vi "XYStage.KIM101.Create Device.vi"(8 "error in (no error)":errorcluster, 11 "SerialNumber":string="97000001") -> (0 "error out":errorcluster, 2 "Device":refnum<k24>, 3 "KCubeInertialMotorControl":refnum<k24>, 5 "CreateDevice Result":bool)   [LabVIEW 2017, in "XYStage.KIM101.lvclass"]
uses:
  XYStage.KIM101.lvclass
  D:/upwork/Laser Measurement Tool/Laser/project/data/Thorlabs.MotionControl.Controls.dll
  data/Thorlabs.MotionControl.Controls.dll
  D:/upwork/Laser Measurement Tool/Laser/project/data/Thorlabs.MotionControl.KCube.InertialMotorCLI.dll
  data/Thorlabs.MotionControl.KCube.InertialMotorCLI.dll
panel:
  in  "KCubeInertialMotorControl":refnum<k24>(container)
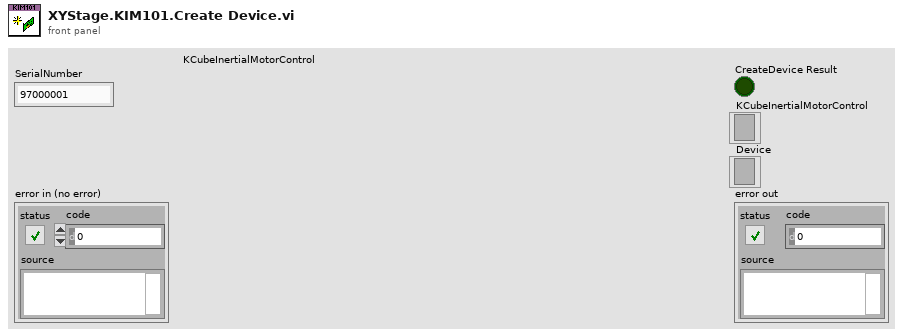
[diagram p1: front panel]
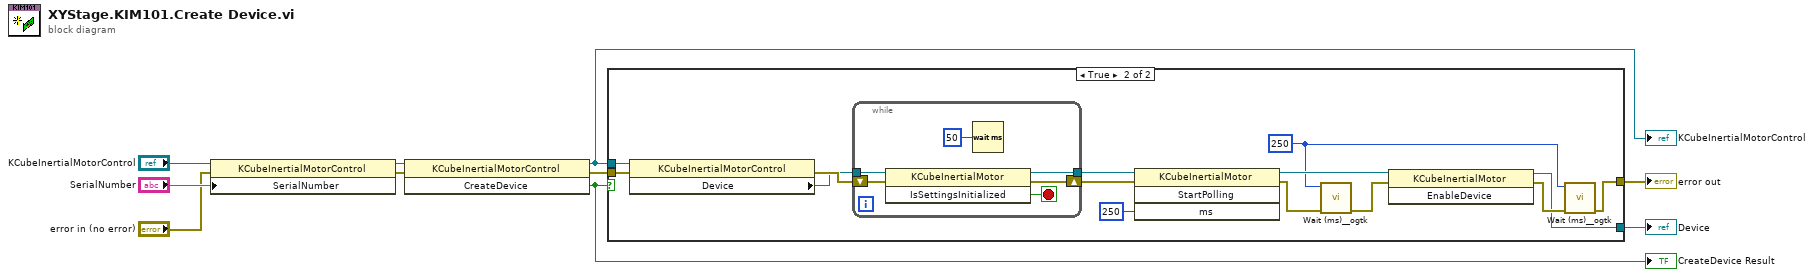
[diagram p0: block diagram]
diagram:
  n1 = property class="KCubeInertialMotorControl"(reference="KCubeInertialMotorControl", error in="error in (no error)", "SerialNumber"="SerialNumber") -> (reference out=w8:refnum<k24>, error out=w7:errorcluster)
  n2 = invoke class="KCubeInertialMotorControl" method="CreateDevice"(reference=w8, error in=w7) -> (reference out=w1:refnum<k24>, error out=w5:errorcluster, "CreateDevice"=w6:bool)  [unwired: 1 in]
  "CreateDevice Result" <- w6
  "KCubeInertialMotorControl" <- w1
  n3 = case shown="True" w6 {
    tunnel: w1 -> [_ w24]
    tunnel: w5 -> [w11 w25]
    tunnel: [_ w12] -> w2
    tunnel: [w11 w14] -> w4
    frame False {
    }
    frame True {
      w13 = u32 250 ("milliseconds to wait")
      n4 = property class="KCubeInertialMotorControl"(reference=w24, error in=w25) -> (error out=w20:errorcluster, "Device"=w19:refnum<k24>)  [unwired: 1 out]
      n5 = while {
        tunnel: [w30] -> w23
        tunnel: w19 -> [w26]
        shift-right: [w27] -> w21
        shift-left: w20 -> [w28]
        stop <- w31 stop-if-true
        n6 = invoke class="KCubeInertialMotor" method="IsSettingsInitialized"(reference=w26, error in=w28) -> (reference out=w30:refnum<k24>, error out=w27:errorcluster, "IsSettingsInitialized"=w31:bool)  [unwired: 1 in]
        n7 = Wait (ms)(milliseconds to wait=u32 50) -> ()  [unwired: 1 out]
      }
      n8 = invoke class="KCubeInertialMotor" method="StartPolling"(reference=w23, error in=w21, "ms"=250) -> (reference out=w18:refnum<k24>, error out=w17:errorcluster)  [unwired: 1 in, 2 out]
      n9 = call <userlib>:"Wait (ms)__ogtk.vi"("error in (no error)"=w17, "milliseconds to wait"=w13) -> ("error out"=w16:errorcluster)  [unwired: 8 in, 1 out]
      n10 = invoke class="KCubeInertialMotor" method="EnableDevice"(reference=w18, error in=w16) -> (reference out=w12:refnum<k24>, error out=w15:errorcluster)  [unwired: 1 in, 1 out]
      n11 = call <userlib>:"Wait (ms)__ogtk.vi"("error in (no error)"=w15, "milliseconds to wait"=w13) -> ("error out"=w14:errorcluster)  [unwired: 8 in, 1 out]
    }
  }
  "error out" <- w4
  "Device" <- w2
